vi "WPI_IMU_ADIS16448_AHRS_Madgwick.vi"(6 "Yaw Axis":enum16{"X", "Y", "Z"}(ring)=enum."Z", 8 "Reset?":bool, 10 "Beta":dbl, 11 "Data":dbl[](array[numeric])) -> (3 "Output":cluster{"Pitch":dbl, "Roll":dbl, "Yaw":dbl})   [LabVIEW 2015, in "Apple Pi Gyro Library.lvlib" / "FRC_ADIS16448_IMU.lvlib"]
uses:
  FRC_ADIS16448_IMU.lvlib
panel:
  out "Quaternion":dbl[](array[numeric])
  out "Pitch":dbl
  out "Roll":dbl
  out "Yaw":dbl
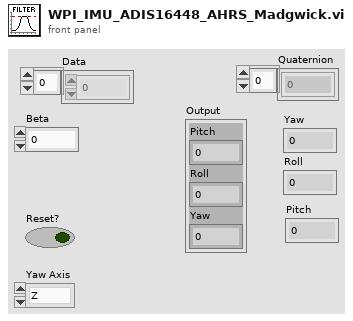
[diagram p1: front panel]
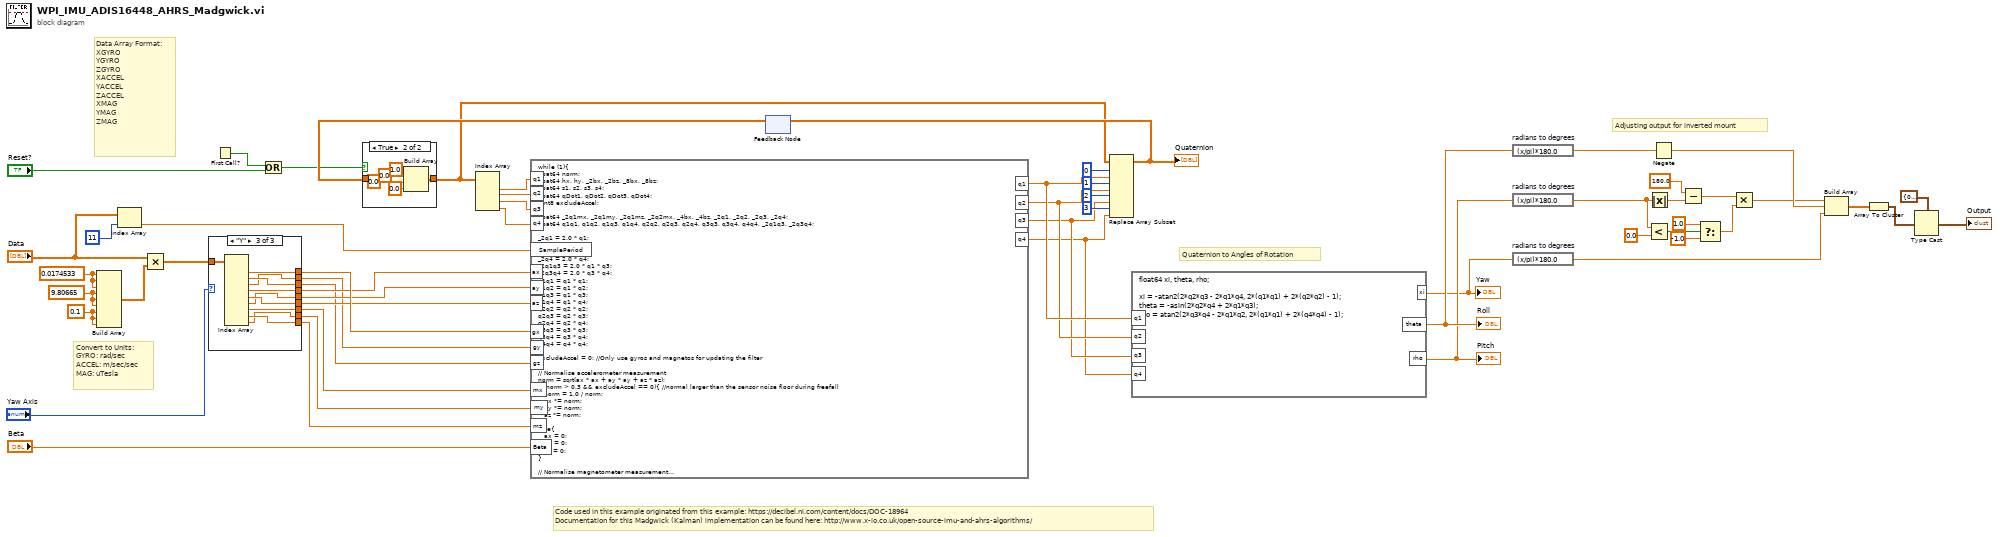
[diagram p0: block diagram]
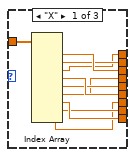
[diagram p2: hidden frame]
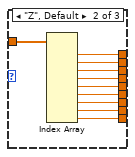
[diagram p3: hidden frame]
diagram:
  w51 = 0.1
  w52 = 9.80665
  w53 = 0.0174533
  # "Code used in this example originated from this example: https://decibel.ni.com/content/docs/DOC-18964\nDocumentation for this Madgwick (Kalman) implementation can be found here: http://www.x-io.co.uk/open-source-imu-and-ahrs-algorithms/"
  # "Quaternion to Angles of Rotation"
  # "Convert to Units:\nGYRO: rad/sec\nACCEL: m/sec/sec\nMAG: uTesla"
  # "Data Array Format:\nXGYRO\nYGYRO\nZGYRO\nXACCEL\nYACCEL\nZACCEL\nXMAG\nYMAG\nZMAG"
  # "Adjusting output for inverted mount"
  n1 = Build Array(w53, w53, w53, w52, w52, w52, w51, w51, w51) -> (w54:dbl[])
  n2 = Index Array(array="Data", index=11) -> (element=w5:dbl)
  n3 = Multiply(x="Data", y=w54) -> (x*y=w50:dbl[])
  n4 = case shown="\"Y\"" "Yaw Axis" {
    tunnel: [w64 w77 w86] -> w57
    tunnel: [w61 w76 w83] -> w56
    tunnel: w50 -> [w67 w75 w87]
    tunnel: [w58 w74 w80] -> w27
    tunnel: [w62 w73 w81] -> w26
    tunnel: [w63 w72 w82] -> w25
    tunnel: [w65 w71 w84] -> w24
    tunnel: [w66 w70 w85] -> w23
    tunnel: [w59 w69 w78] -> w22
    tunnel: [w60 w68 w79] -> w21
    frame "X" {
      n5 = Index Array(array=w67) -> (element #1=w66:dbl, element #2=w65:dbl, element #3=w64:dbl, element #4=w63:dbl, element #5=w62:dbl, element #6=w61:dbl, element #7=w60:dbl, element #8=w59:dbl, element #9=w58:dbl)  [unwired: 9 in]
    }
    frame "Z", Default {
      n6 = Index Array(array=w75) -> (element #1=w77:dbl, element #2=w71:dbl, element #3=w70:dbl, element #4=w76:dbl, element #5=w73:dbl, element #6=w72:dbl, element #7=w74:dbl, element #8=w69:dbl, element #9=w68:dbl)  [unwired: 9 in]
    }
    frame "Y" {
      n7 = Index Array(array=w87) -> (element #1=w86:dbl, element #2=w85:dbl, element #3=w84:dbl, element #4=w83:dbl, element #5=w82:dbl, element #6=w81:dbl, element #7=w80:dbl, element #8=w79:dbl, element #9=w78:dbl)  [unwired: 9 in]
    }
  }
  n8 = First Call?() -> (First Call?: T/F=w33:bool)
  n9 = Or(x=w33, y="Reset?") -> (x .or. y?=w34:bool)
  n10 = feedback #1() -> (w36:dbl[])  [unwired: 1 in]
  n11 = case shown="True" w34 {
    tunnel: w36 -> [w88 _]
    tunnel: [w88 w89] -> w35
    frame False {
    }
    frame True {
      n12 = Build Array(1.0 ("element"), 0.0 ("element"), 0.0 ("element"), 0.0 ("element")) -> (w89:dbl[])
    }
  }
  n13 = Index Array(array=w35) -> (element #1=w49:dbl, element #2=w48:dbl, element #3=w47:dbl, element #4=w46:dbl)  [unwired: 4 in]
  n14 = formula code="while (1){\nfloat64 norm;\nfloat64 hx, hy, _2bx, _2bz, _8bx, _8bz;\nfloat64 s1, s2, s3, s4;\nfloat64 qDot1, qDot2, qDot3, qDot4;\nuInt8 excludeAccel;\n\nfloat64 _2q1mx, _2q1my, _2q1mz, _2q2mx, _4bx, _4bz, _2q1, _2q2, _2q3, _2q4;\nfloat64 q1q1, q1q2, q1q3, q1q4, q2q2, q2q3, q2q4, q3q3, q3q4, q4q4, _2q1q3, _2q3q4;\n\n_2q1 = 2.0 * q1;\n_2q2 = 2.0 * q2;\n_2q3 = 2.0 * q3;\n_2q4 = 2.0 * q4;\n_2q1q3 = 2.0 * q1 * q3;\n_2q3q4 = 2.0 * q3 * q4;\nq1q1 = q1 * q1;\nq1q2 = q1 * q2;\nq1q3 = q1 * q3;\nq1q4 = q1 * q4;\nq2q2 = q2 * q2;\nq2q3 = q2 * q3;\nq2q4 = q2 * q4;\nq3q3 = q3 * q3;\nq3q4 = q3 * q4;\nq4q4 = q4 * q4;\n\nexcludeAccel = 0; //Only use gyros and magnetos for updating the filter\n\n// Normalise accelerometer measurement\nnorm = sqrt(ax * ax + ay * ay + az * az);\nif (norm > 0.3 && excludeAccel == 0){ //normal larger than the sensor noise floor during freefall\n   norm = 1.0 / norm; \n   ax *= norm;\n   ay *= norm;\n   az *= norm;\n}\nelse{\n   ax = 0;\n   ay = 0;\n   az = 0;\n}\n\n// Normalise magnetometer measurement\nnorm = sqrt(mx * mx + my * my + mz * mz);\nif (norm > 0.0){\n   norm = 1.0 / norm;\n   mx *= norm;\n   my *= norm;\n   mz *= norm;\n}\nelse{\n  break; //something is wrong with the magneto readouts\n}\n\n// Reference direction of Earth's magnetic field\n_2q1mx = 2 * q1 * mx;\n_2q1my = 2 * q1 * my;\n_2q1mz = 2 * q1 * mz;\n_2q2mx = 2 * q2 * mx;\n\nhx = mx * q1q1 - _2q1my * q4 + _2q1mz * q3 + mx * q2q2 + _2q2 * my * q3 + _2q2 * mz * q4 - mx * q3q3 - mx * q4q4;\nhy = _2q1mx * q4 + my * q1q1 - _2q1mz * q2 + _2q2mx * q3 - my * q2q2 + my * q3q3 + _2q3 * mz * q4 - my * q4q4;\n_2bx = sqrt(hx * hx + hy * hy);\n_2bz = -_2q1mx * q3 + _2q1my * q2 + mz * q1q1 + _2q2mx * q4 - mz * q2q2 + _2q3 * my * q4 - mz * q3q3 + mz * q4q4;\n_4bx = 2.0 * _2bx;\n_4bz = 2.0 * _2bz;\n_8bx = 2.0 * _4bx;\n_8bz = 2.0 * _4bz;\n\n// Gradient descent algorithm corrective step\ns1 = -_2q3 * (2.0 * q2q4 - _2q1q3 - ax) + _2q2 * (2.0 * q1q2 + _2q3q4 - ay) - _4bz * q3 * (_4bx * (0.5 - q3q3 - q4q4) + _4bz * (q2q4 - q1q3) - mx) + (-_4bx * q4 + _4bz * q2) * (_4bx * (q2q3 - q1q4) + _4bz * (q1q2 + q3q4) - my) + _4bx * q3 * (_4bx * (q1q3 + q2q4) + _4bz * (0.5 - q2q2 - q3q3) - mz);\ns2 = _2q4 * (2.0 * q2q4 - _2q1q3 - ax) + _2q1 * (2.0 * q1q2 + _2q3q4 - ay) - 4.0 * q2 * (1.0 - 2.0 * q2q2 - 2.0 * q3q3 - az) + _4bz * q4 * (_4bx * (0.5 - q3q3 - q4q4) + _4bz * (q2q4 - q1q3) - mx) + (_4bx * q3 + _4bz * q1) * (_4bx * (q2q3 - q1q4) + _4bz * (q1q2 + q3q4) - my) + (_4bx * q4 - _8bz * q2) * (_4bx * (q1q3 + q2q4) + _4bz * (0.5 - q2q2 - q3q3) - mz);\ns3 = -_2q1 * (2.0 * q2q4 - _2q1q3 - ax) + _2q4 * (2.0 * q1q2 + _2q3q4 - ay) - 4.0 * q3 * (1.0 - 2.0 * q2q2 - 2.0 * q3q3 - az) + (-_8bx * q3 - _4bz * q1) * (_4bx * (0.5 - q3q3 - q4q4) + _4bz * (q2q4 - q1q3) - mx) + (_4bx * q2 + _4bz * q4) * (_4bx * (q2q3 - q1q4) + _4bz * (q1q2 + q3q4) - my) + (_4bx * q1 - _8bz * q3) * (_4bx * (q1q3 + q2q4) + _4bz * (0.5 - q2q2 - q3q3) - mz);\ns4 = _2q2 * (2.0 * q2q4 - _2q1q3 - ax) + _2q3 * (2.0 * q1q2 + _2q3q4 - ay) + (-_8bx * q4 + _4bz * q2) * (_4bx * (0.5 - q3q3 - q4q4) + _4bz * (q2q4 - q1q3) - mx) + (-_4bx * q1 + _4bz * q3) * (_4bx * (q2q3 - q1q4) + _4bz * (q1q2 + q3q4) - my) + _4bx * q2 * (_4bx * (q1q3 + q2q4) + _4bz * (0.5 - q2q2 - q3q3) - mz);\n\nnorm = sqrt(s1 * s1 + s2 * s2 + s3 * s3 + s4 * s4);\nif (norm > 0.0){\n   norm = 1.0 / norm;  //normalise gradient step\n   s1 *= norm;\n   s2 *= norm;\n   s3 *= norm;\n   s4 *= norm;\n}\nelse{\n   break;\n}\n\n// Compute rate of change of quaternion\nqDot1 = 0.5 * (-q2 * gx - q3 * gy - q4 * gz) - Beta * s1;\nqDot2 = 0.5 * (q1 * gx + q3 * gz - q4 * gy) - Beta * s2;\nqDot3 = 0.5 * (q1 * gy - q2 * gz + q4 * gx) - Beta * s3;\nqDot4 = 0.5 * (q1 * gz + q2 * gy - q3 * gx) - Beta * s4;\n\n// Integrate to yield quaternion\nq1 += qDot1 * SamplePeriod;\nq2 += qDot2 * SamplePeriod;\nq3 += qDot3 * SamplePeriod;\nq4 += qDot4 * SamplePeriod;\n\nnorm = sqrt(q1 * q1 + q2 * q2 + q3 * q3 + q4 * q4);\nif (norm > 0.0){\n   norm = 1.0 / norm;  //normalise quaternion\n   q1 = q1 * norm;\n   q2 = q2 * norm;\n   q3 = q3 * norm;\n   q4 = q4 * norm;\n}\nbreak;\n}"("q1"=w49, "gx"=w57, "gy"=w24, "gz"=w23, "ax"=w56, "ay"=w26, "az"=w25, "mx"=w27, "my"=w22, "mz"=w21, "SamplePeriod"=w5, "Beta"="Beta", "q2"=w48, "q3"=w47, "q4"=w46) -> ("q1"=w40:dbl, "q2"=w39:dbl, "q3"=w38:dbl, "q4"=w37:dbl)
  n15 = Replace Array Subset(array=w35, new element #1=w40, index #1=0 ("index"), new element #2=w39, index #2=1 ("index"), new element #3=w38, index #3=2 ("index"), new element #4=w37, index #4=3 ("index")) -> (w41:dbl[])
  "Quaternion" <- w41
  n16 = feedback-in #1(w41) -> ()
  n17 = formula code="float64 xi, theta, rho;\n\nxi = -atan2(2*q2*q3 - 2*q1*q4, 2*(q1*q1) + 2*(q2*q2) - 1);\ntheta = -asin(2*q2*q4 + 2*q1*q3);\nrho = atan2(2*q3*q4 - 2*q1*q2, 2*(q1*q1) + 2*(q4*q4) - 1);"("q1"=w40, "q2"=w39, "q3"=w38, "q4"=w37) -> ("xi"=w29:dbl, "theta"=w31:dbl, "rho"=w30:dbl)
  "Yaw" <- w29
  "Roll" <- w31
  "Pitch" <- w30
  n18 = expression code="(x/pi)*180.0" "radians to degrees"(w31) -> (w11:dbl)
  n19 = expression code="(x/pi)*180.0" "radians to degrees"(w30) -> (w18:dbl)
  n20 = expression code="(x/pi)*180.0" "radians to degrees"(w29) -> (w28:dbl)
  n21 = Less?(x=w18, y=0.0) -> (x < y?=w16:bool)
  n22 = Absolute Value(x=w18) -> (abs(x)=w20:dbl)
  n23 = Negate(x=w11) -> (-x=w10:dbl)
  n24 = Subtract(x=180.0 ("y"), y=w20) -> (x-y=w13:dbl)
  n25 = Select(t=1.0, s=w16, f=-1.0) -> (s? t:f=w12:dbl)
  n26 = Multiply(x=w13, y=w12) -> (x*y=w9:dbl)
  n27 = Build Array(w9, w10, w28) -> (w2:dbl[])
  n28 = Array To Cluster(array=w2) -> (cluster=w3:cluster{"[0]":dbl, "[1]":dbl, "[2]":dbl})
  n29 = Type Cast(type=cluster{"Pitch":dbl, "Roll":dbl, "Yaw":dbl} {"Pitch"=0.0, "Roll"=0.0, "Yaw"=0.0} ("IMU AHRS"), x=w3) -> (*(type *) &x=→"Output":cluster{"Pitch":dbl, "Roll":dbl, "Yaw":dbl})
